vi "Tracking_SubVI-3.vi"(7 "[IN] Control Parameters":T4, 8 "error IN":errorcluster, 9 "[IN] Before-After Tracks":T3, 11 "[IN] Movie Values":T2 {"Particle Fil Setups"."Type of particle filter"."Measurement Parameter" items=["Center of Mass X", "Center of Mass Y", "First Pixel X", "First Pixel Y", "Bounding Rect Left", "Bounding Rect Top", "Bounding Rect Right", "Bounding Rect Bottom", "Max Feret Diameter Start X", "Max Feret Diameter Start Y", "Max Feret Diameter End X", "Max Feret Diameter End Y", "Max Horiz. Segment Length Left", "Max Horiz. Segment Length Right", "Max Horiz. Segment Length Row", "-", "Bounding Rect Width", "Bounding Rect Height", "Bounding Rect Diagonal", "Perimeter", "Convex Hull Perimeter", "Holes' Perimeter", "Max Feret Diameter", "Equivalent Ellipse Major Axis", "Equivalent Ellipse Minor Axis", "Equivalent Ellipse Minor Axis (Feret)", "Equivalent Rect Long Side", "Equivalent Rect Short Side", "Equivalent Rect Diagonal", "Equivalent Rect Short Side (Feret)", "Average Horiz. Segment Length", "Average Vert. Segment Length", "Hydraulic Radius", "Waddel Disk Diameter", "-", "Area", "Holes' Area", "Particle & Holes' Area", "Convex Hull Area", "Image Area", "-", "Number of Holes", "Number of Horiz. Segments", "Number of Vert. Segments", "-", "Orientation", "Max Feret Diameter Orientation", "-", "% Area/Image Area", "% Area/(Particle & Holes' Area)", "Ratio of Equivalent Ellipse Axes", "Ratio of Equivalent Rect Sides", "-", "Elongation Factor", "Compactness Factor", "Heywood Circularity Factor", "Type Factor", "-", "Sum X", "Sum Y", "Sum XX", "Sum XY", "Sum YY", "Sum XXX", "Sum XXY", "Sum XYY", "Sum YYY", "-", "Moment of Inertia XX", "Moment of Inertia XY", "Moment of Inertia YY", "Moment of Inertia XXX", "Moment of Inertia XXY", "Moment of Inertia XYY", "Moment of Inertia YYY", "Norm. Moment of Inertia XX", "Norm. Moment of Inertia XY", "Norm. Moment of Inertia YY", "Norm. Moment of Inertia XXX", "Norm. Moment of Inertia XXY", "Norm. Moment of Inertia XYY", "Norm. Moment of Inertia YYY", "Hu Moment 1", "Hu Moment 2", "Hu Moment 3", "Hu Moment 4", "Hu Moment 5", "Hu Moment 6", "Hu Moment 7"]}) -> (0 "error OUT":errorcluster, 1 "[OUT] Before-After Tracks":T3, 3 "[OUT] Tracking Movie Values":T2 {"Particle Fil Setups"."Type of particle filter"."Measurement Parameter" items=["Center of Mass X", "Center of Mass Y", "First Pixel X", "First Pixel Y", "Bounding Rect Left", "Bounding Rect Top", "Bounding Rect Right", "Bounding Rect Bottom", "Max Feret Diameter Start X", "Max Feret Diameter Start Y", "Max Feret Diameter End X", "Max Feret Diameter End Y", "Max Horiz. Segment Length Left", "Max Horiz. Segment Length Right", "Max Horiz. Segment Length Row", "-", "Bounding Rect Width", "Bounding Rect Height", "Bounding Rect Diagonal", "Perimeter", "Convex Hull Perimeter", "Holes' Perimeter", "Max Feret Diameter", "Equivalent Ellipse Major Axis", "Equivalent Ellipse Minor Axis", "Equivalent Ellipse Minor Axis (Feret)", "Equivalent Rect Long Side", "Equivalent Rect Short Side", "Equivalent Rect Diagonal", "Equivalent Rect Short Side (Feret)", "Average Horiz. Segment Length", "Average Vert. Segment Length", "Hydraulic Radius", "Waddel Disk Diameter", "-", "Area", "Holes' Area", "Particle & Holes' Area", "Convex Hull Area", "Image Area", "-", "Number of Holes", "Number of Horiz. Segments", "Number of Vert. Segments", "-", "Orientation", "Max Feret Diameter Orientation", "-", "% Area/Image Area", "% Area/(Particle & Holes' Area)", "Ratio of Equivalent Ellipse Axes", "Ratio of Equivalent Rect Sides", "-", "Elongation Factor", "Compactness Factor", "Heywood Circularity Factor", "Type Factor", "-", "Sum X", "Sum Y", "Sum XX", "Sum XY", "Sum YY", "Sum XXX", "Sum XXY", "Sum XYY", "Sum YYY", "-", "Moment of Inertia XX", "Moment of Inertia XY", "Moment of Inertia YY", "Moment of Inertia XXX", "Moment of Inertia XXY", "Moment of Inertia XYY", "Moment of Inertia YYY", "Norm. Moment of Inertia XX", "Norm. Moment of Inertia XY", "Norm. Moment of Inertia YY", "Norm. Moment of Inertia XXX", "Norm. Moment of Inertia XXY", "Norm. Moment of Inertia XYY", "Norm. Moment of Inertia YYY", "Hu Moment 1", "Hu Moment 2", "Hu Moment 3", "Hu Moment 4", "Hu Moment 5", "Hu Moment 6", "Hu Moment 7"]}, 4 "[OUT] # Displ after Filtration":i32, 6 "[OUT] # Displ w/t Filters":i32)   [LabVIEW 2013]
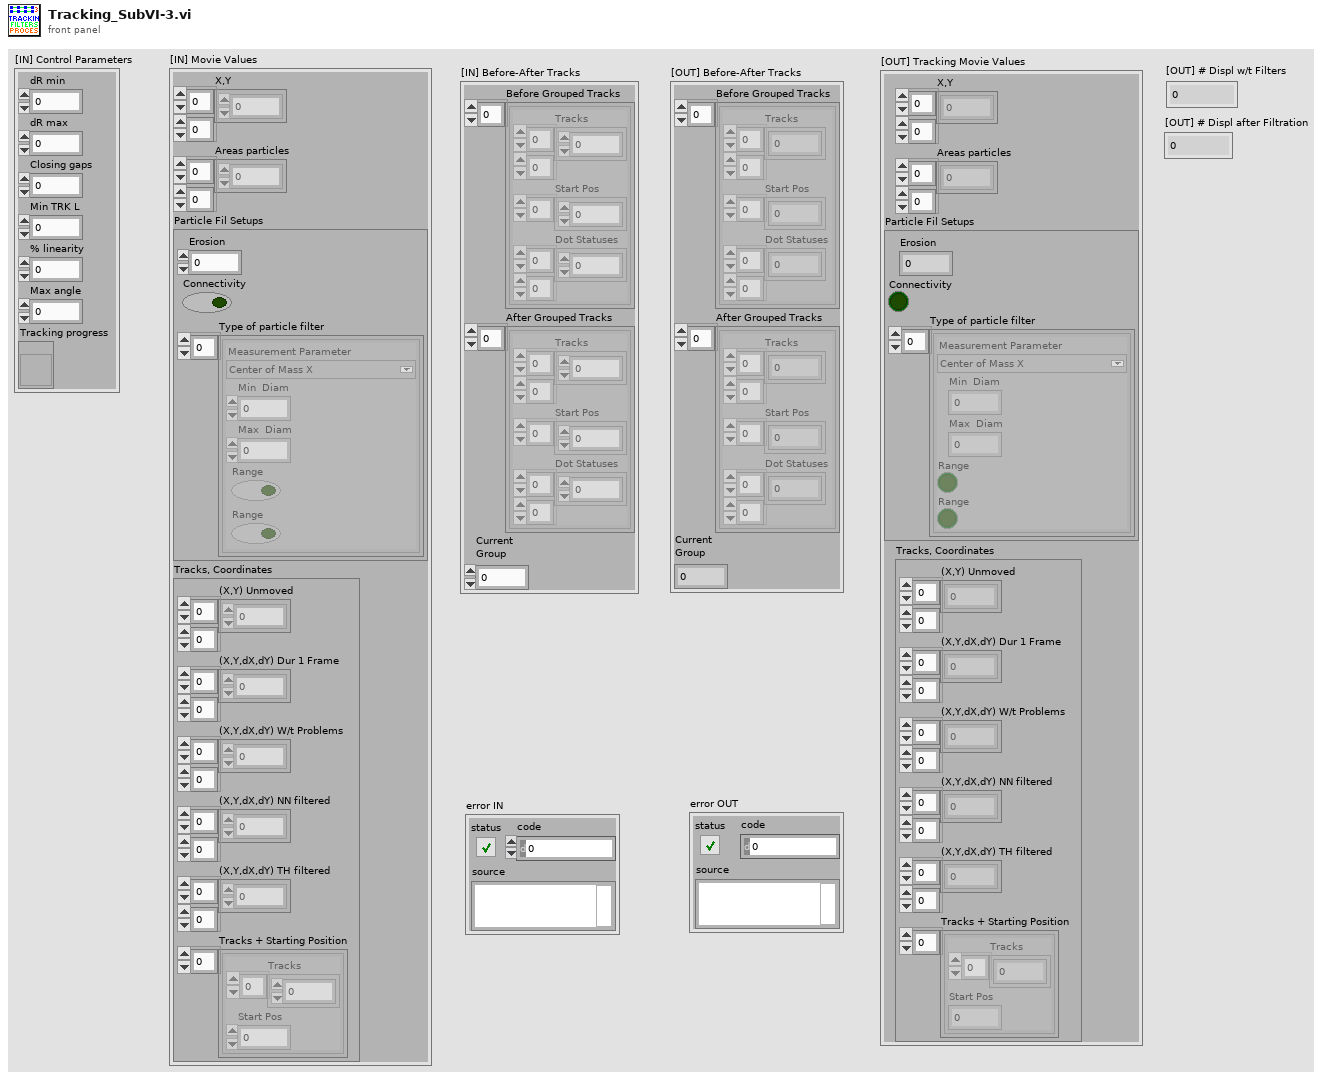
[diagram p1: front panel]
types:
  T1 = typedef "Particle Parameters" = i32
  T2 = cluster{"X,Y":dbl[][], "Areas particles":dbl[][], "Particle Fil Setups":cluster{"Erosion":i32, "Connectivity ":bool, "Type of particle filter":cluster{"Measurement Parameter":T1, "Min  Diam":dbl, "Max  Diam":dbl, "Range":bool, "Range":bool}[]}, "Tracks, Coordinates":cluster{"(X,Y) Unmoved":dbl[][], "(X,Y,dX,dY) Dur 1 Frame":dbl[][], "(X,Y,dX,dY) W/t Problems":dbl[][], "(X,Y,dX,dY) NN filtered":dbl[][], "(X,Y,dX,dY) TH filtered":dbl[][], "Tracks + Starting Position":cluster{"Tracks":dbl[], "Start Pos":i32}[]}}
  T3 = cluster{"Before Grouped Tracks":cluster{"Tracks":dbl[][], "Start Pos":i32[], "Dot Statuses":i16[][]}[], "After Grouped Tracks":cluster{"Tracks":dbl[][], "Start Pos":i32[], "Dot Statuses":i16[][]}[], "Current\nGroup":i32}
  T4 = cluster{"dR min ":dbl, "dR max ":dbl, "Closing gaps":i32, "Min TRK L":i32, "% linearity":i32, "Max angle":dbl, "Tracking progress":refnum<vi>}
  T5 = cluster{"Erosion":i32, "Connectivity ":bool, "Type of particle filter":cluster{"Measurement Parameter":T1, "Min  Diam":dbl, "Max  Diam":dbl, "Range":bool, "Range":bool}[]}
  T6 = cluster{"(X,Y) Unmoved":dbl[][], "(X,Y,dX,dY) Dur 1 Frame":dbl[][], "(X,Y,dX,dY) W/t Problems":dbl[][], "(X,Y,dX,dY) NN filtered":dbl[][], "(X,Y,dX,dY) TH filtered":dbl[][], "Tracks + Starting Position":cluster{"Tracks":dbl[], "Start Pos":i32}[]}
  T7 = cluster{"Tracks W/T Problems":dbl[], "Start Pos":i32}[]
  T8 = cluster{"Tracks":dbl[][], "Start Pos":i32[], "Dot Statuses":i16[][]}[]
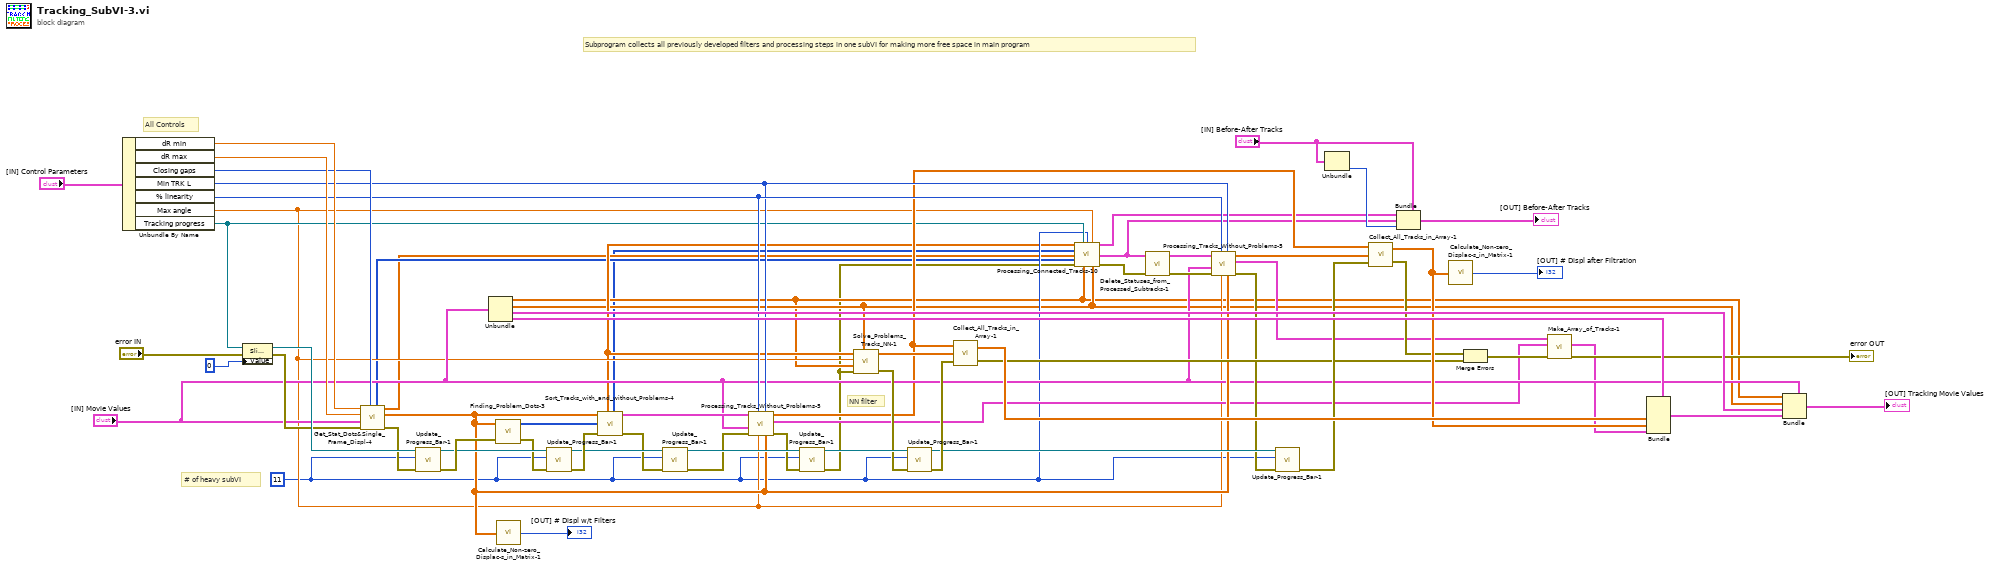
[diagram p0: block diagram]
diagram:
  w11 = 11 ("[IN] Number of SubVI")
  # "Subprogram collects all previously developed filters and processing steps in one subVI for making more free space in main program"
  # "NN filter"
  # "# of heavy subVI"
  # "All Controls"
  n1 = Unbundle By Name("[IN] Control Parameters") -> ("dR min"=w36:dbl, "dR max"=w35:dbl, "Closing gaps"=w33:i32, "Min TRK L"=w26:i32, "% linearity"=w27:i32, "Max angle"=w12:dbl, "Tracking progress"=w13:refnum<vi>)
  n2 = property on="Property Node" class="Slide (strict)"(reference=w13, error in="error IN", "Value"=u8 0) -> (reference out=w38:refnum<vi>, error out=w34:errorcluster)
  n3 = call "Get_Stat_Dots&Single_Frame_Displ-4.vi"("Closing gaps"=w33, "[IN] error"=w34, "[IN] Movie Values"="[IN] Movie Values", "dR max"=w35, "dR min"=w36) -> ("error OUT"=w32:errorcluster, "[OUT] Displacements \nwith Length >1 Frame"=w24:dbl[][], "[OUT] (X,Y) Poten-\ntially Moving"=w2:dbl[][], "[OUT] Dot matrix after using \nsome filters which contains \ndots with increased statuses"=w3:i16[][])  [unwired: 3 out]
  n4 = call "Update_Progress_Bar-1.vi"("error IN"=w32, "[IN] Number of SubVI"=w11, "[IN] Tracking progress"=w38) -> ("error OUT"=w64:errorcluster, "[OUT] Tracking progress"=w63:refnum<vi>)  [unwired: 3 in]
  n5 = Unbundle("[IN] Movie Values") -> ("X,Y"=w5:dbl[][], "Areas particles"=w6:dbl[][], "Particle Fil Setups"=w57:T5, "Tracks, Coordinates"=w56:T6)
  n6 = call "Finding_Problem_Dots-3.vi"("error IN"=w64, "[IN] Frame-to-frame displ"=w24) -> ("error OUT"=w62:errorcluster, "[OUT] Dot matrix"=w65:i16[][])  [unwired: 2 in]
  n7 = call "Calculate_Non-zero_Displac-s_in_Matrix-1.vi"("[IN] Displacements \nFrm-to-Frm In Cols"=w24) -> ("[OUT] Number of \n(X,Y,dX,dY) displ-s"=→"[OUT] # Displ w/t Filters":i32)
  n8 = call "Update_Progress_Bar-1.vi"("error IN"=w62, "[IN] Number of SubVI"=w11, "[IN] Tracking progress"=w63) -> ("error OUT"=w61:errorcluster, "[OUT] Tracking progress"=w60:refnum<vi>)  [unwired: 3 in]
  n9 = call "Sort_Tracks_with_and_without_Problems-4.vi"("error IN"=w61, "[IN] Dot matrix"=w65, "[IN}Frame-to-frame displ"=w24) -> ("error OUT"=w59:errorcluster, "[OUT] Tracks w/t Problems"=w31:T7, "[OUT] Filtered Dot Matrix"=w1:i16[][], "[OUT] Displacements with problems\nCollected in Columns (as raw displ)"=w10:dbl[][])  [unwired: 2 in, 1 out]
  n10 = call "Update_Progress_Bar-1.vi"("error IN"=w59, "[IN] Number of SubVI"=w11, "[IN] Tracking progress"=w60) -> ("error OUT"=w30:errorcluster, "[OUT] Tracking progress"=w54:refnum<vi>)  [unwired: 3 in]
  n11 = call "Processing_Tracks_Without_Problems-5.vi"("[IN] Original Displacements\nRecorded in Frames (Columns)"=w24, "[IN] Min TRK L"=w26, "[IN] Max angle between \ntwo displacements"=w12, "[IN] % linearity"=w27, "error IN"=w30, "[IN] Movie Values"="[IN] Movie Values", "[IN] Tracks w/t Problems"=w31) -> ("error OUT"=w29:errorcluster, "[OUT] Filtered Tracks"=w15:T7, "[OUT] Frame-to-Frame Displacements\n Extract From Tracks"=w16:dbl[][])  [unwired: 2 in]
  n12 = call "Update_Progress_Bar-1.vi"("error IN"=w29, "[IN] Number of SubVI"=w11, "[IN] Tracking progress"=w54) -> ("error OUT"=w4:errorcluster, "[OUT] Tracking progress"=w53:refnum<vi>)  [unwired: 3 in]
  n13 = call "Solve_Problems_Tracks_NN-1.vi"("Tracks (unsorted, cols)"=w10, "Max angle"=w12, "X,Y"=w5, "error IN"=w4, "Areas"=w6) -> ("Tracks (X,Y,dX,dY)"=w50:dbl[][], "error OUT"=w52:errorcluster)  [unwired: 1 out]
  n14 = call "Update_Progress_Bar-1.vi"("error IN"=w52, "[IN] Number of SubVI"=w11, "[IN] Tracking progress"=w53) -> ("error OUT"=w51:errorcluster, "[OUT] Tracking progress"=w47:refnum<vi>)  [unwired: 3 in]
  n15 = call "Collect_All_Tracks_in_Array-1.vi"("error in"=w51, "Tracks(Frames) #2"=w50, "Tracks(Frames) #1"=w16) -> ("error out"=w44:errorcluster, "[OUT] Collected Tracks"=w49:dbl[][])
  n16 = call "Processing_Connected_Tracks-10.vi"("[IN] Unsorted \nProblem Tracks"=w10, "[IN] Tracking progress"=w13, "[IN] Number of SubVI"=w11, "[IN] Max angle"=w12, "[IN] Dot matrix \nfor moving points\n(splitted tracks)"=w1, "[IN] Potentially\nMoving (X,Y)"=w2, "[IN] Dot matrix with \nstatuses for potentially \nmoving dots"=w3, "error IN"=w4, "[IN] Primary \n(X,Y) Detected"=w5, "[IN] Areas particles\nPrimary Detected"=w6) -> ("[OUT] Before Processing Tracks"=w9:T8, "[OUT] Processed Tracks"=w8:T8, "error OUT"=w7:errorcluster)  [unwired: 3 in]
  n17 = call "Delete_Statuses_from_Processed_Subtracks-1.vi"("error IN"=w7, "[IN] Processed Tracks"=w8) -> ("error OUT"=w25:errorcluster, "[OUT] Tracks"=w28:cluster{"Track":dbl[], "Start Pos":i32}[])  [unwired: 4 in]
  n18 = call "Processing_Tracks_Without_Problems-5.vi"("[IN] Original Displacements\nRecorded in Frames (Columns)"=w24, "[IN] Min TRK L"=w26, "[IN] Max angle between \ntwo displacements"=w12, "[IN] % linearity"=w27, "error IN"=w25, "[IN] Movie Values"="[IN] Movie Values", "[IN] Tracks w/t Problems"=w28) -> ("error OUT"=w23:errorcluster, "[OUT] Filtered Tracks"=w17:T7, "[OUT] Frame-to-Frame Displacements\n Extract From Tracks"=w22:dbl[][])  [unwired: 2 in]
  n19 = call "Update_Progress_Bar-1.vi"("error IN"=w23, "[IN] Number of SubVI"=w11, "[IN] Tracking progress"=w47) -> ("error OUT"=w46:errorcluster)  [unwired: 3 in, 1 out]
  n20 = Unbundle("[IN] Before-After Tracks") -> ("Current\nGroup"=w41:i32)  [unwired: 2 out]
  n21 = call "Collect_All_Tracks_in_Array-1.vi"("error in"=w46, "Tracks(Frames) #2"=w22, "Tracks(Frames) #1"=w16) -> ("error out"=w43:errorcluster, "[OUT] Collected Tracks"=w45:dbl[][])
  n22 = Bundle(cluster="[IN] Before-After Tracks", "Before Grouped Tracks"=w9, "After Grouped Tracks"=w8, "Current\nGroup"=w41) -> (→"[OUT] Before-After Tracks":T3)
  n23 = call "Calculate_Non-zero_Displac-s_in_Matrix-1.vi"("[IN] Displacements \nFrm-to-Frm In Cols"=w45) -> ("[OUT] Number of \n(X,Y,dX,dY) displ-s"=→"[OUT] # Displ after Filtration":i32)
  n24 = Merge Errors(w43, w44) -> (w19:errorcluster)
  n25 = call "Make_Array_of_Tracks-1.vi"("error IN"=w19, "[IN] Filtered Tracks w/t Problems"=w15, "[IN] Filtered Tracks with Problems"=w17) -> ("error OUT"=→"error OUT":errorcluster, "[OUT] Array of tracks"=w14:cluster{"Tracks":dbl[], "Start Pos":i32}[])  [unwired: 3 in]
  n26 = Bundle(cluster=w56, "(X,Y,dX,dY) NN filtered"=w49, "(X,Y,dX,dY) TH filtered"=w45, "Tracks + Starting Position"=w14) -> (w55:T6)  [unwired: 3 in]
  n27 = Bundle(cluster="[IN] Movie Values", "X,Y"=w5, "Areas particles"=w6, "Particle Fil Setups"=w57, "Tracks, Coordinates"=w55) -> (→"[OUT] Tracking Movie Values":T2)
